vi "Lithographify_funnel_rec.vi"(5 "Data In":cluster{string, cluster{"X":dbl, "Y":dbl}[]}, 7 "Direction":u16, 9 "Speed (µm/s)":T2={"Schedule"=enum."Constant", "Settings"=variant(dbl 0.0)}, 11 "Voltage (V)":T2={"Schedule"=enum."Constant", "Settings"=variant(dbl 0.0)}, 12 "Set Resistance":T1=enum."1G ohm", 13 "Enabled":bool) -> (4 "Lithography Data":T4={"Name"="", "Litho"=[], "Set Resistance"=enum."1G ohm"})   [LabVIEW 2020]
doc: "This VI calculates the lithography data of one pattern and organizes it appropriately."
uses:
  <userlib>/LevyLab/Relay Box/Type_defs/Resistor--enum.ctl
  typedefs/Voltage - cluster.ctl
  typedefs/Schedule - enum.ctl
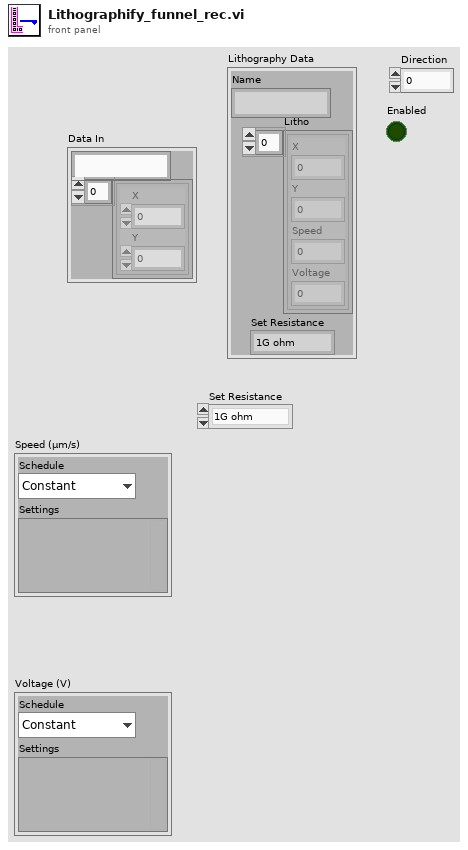
[diagram p1: front panel]
types:
  T1 = typedef "Resistor--enum.ctl" = enum16{"open", "discharge tip", "0 ohms", "100k ohm", "10M ohm", "1G ohm"}
  T2 = typedef "Voltage - cluster.ctl" = cluster{"Schedule":T3, "Settings":variant}
  T3 = typedef "Schedule - enum.ctl" = enum16{"Constant", "Ramp", "Fn. Generator", "Formula"}
  T4 = cluster{"Name":string, "Litho":cluster{"X":dbl, "Y":dbl, "Speed":dbl, "Voltage":dbl}[], "Set Resistance":T1}
  T5 = cluster{"X":dbl, "Y":dbl, "Speed":dbl, "Voltage":dbl}[]
  T6 = cluster{"X":dbl, "Y":dbl, "Speed":dbl, "Voltage":dbl}
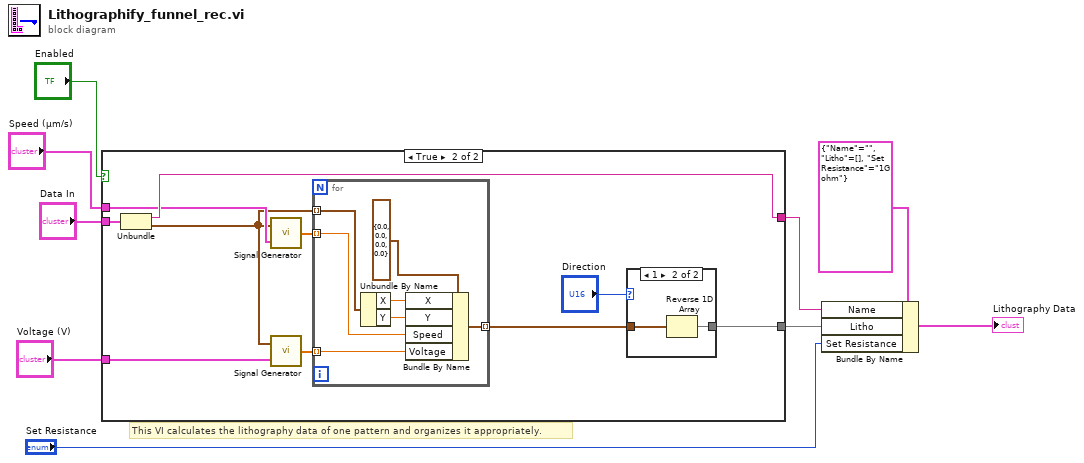
[diagram p0: block diagram]
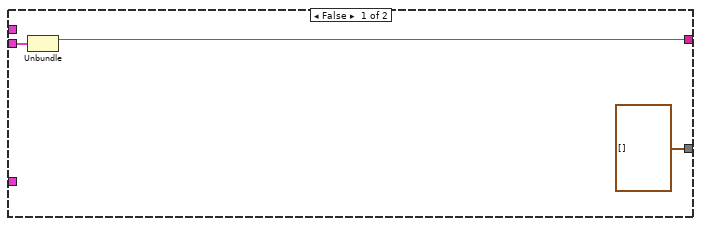
[diagram p2: hidden frame]
diagram:
  # "This VI calculates the lithography data of one pattern and organizes it appropriately."
  n1 = case shown="True" "Enabled" {
    tunnel: [w11 w22] -> w9
    tunnel: "Data In" -> [w12 w21]
    tunnel: "Voltage (V)" -> [_ w18]
    tunnel: "Speed (µm/s)" -> [_ w17]
    tunnel: [T5 [] w15] -> w3
    frame False {
      n2 = Unbundle(w12) -> (w11:string)  [unwired: 1 out]
    }
    frame True {
      n3 = Unbundle(w21) -> (w22:string, w13:cluster{"X":dbl, "Y":dbl}[])
      n4 = call "Signal Generator.vi"("Signal Properties"=w17, "Points"=w13) -> ("Signal"=w19:dbl[])
      n5 = call "Signal Generator.vi"("Signal Properties"=w18, "Points"=w13) -> ("Signal"=w20:dbl[])
      n6 = for {
        tunnel: w19 -> [w28] mode=indexing
        tunnel: w20 -> [w27] mode=indexing
        tunnel: w13 -> [w30] mode=indexing
        tunnel: [w26] -> w16 mode=indexing
        n7 = Unbundle By Name(w30) -> ("X"=w31:dbl, "Y"=w29:dbl)
        n8 = Bundle By Name(cluster=T6 {"X"=0.0, "Y"=0.0, "Speed"=0.0, "Voltage"=0.0} ("Litho Point"), "X"=w31, "Y"=w29, "Speed"=w28, "Voltage"=w27) -> (w26:T6)
      }
      n9 = case shown="1" "Direction" {
        tunnel: w16 -> [w23 w25]
        tunnel: [w23 w24] -> w15
        frame 0, Default {
        }
        frame 1 {
          n10 = Reverse 1D Array(array=w25) -> (reversed array=w24:T5)
        }
      }
    }
  }
  n11 = Bundle By Name(cluster=T4 {"Name"="", "Litho"=[], "Set Resistance"=enum."1G ohm"} ("Lithography Data"), "Name"=w9, "Litho"=w3, "Set Resistance"="Set Resistance") -> (→"Lithography Data":T4)
